vi "AB_Engine_Detect_Additional_Dependencies.vi"(1 "ContextForBuild in":refnum<vi>, 5 "collect dependencies?":bool, 9 "Dependencies in":T1[](array[typedef]), 11 "error in (no error)":errorcluster) -> (10 "Dependencies out":T1[](array[typedef]), 15 "error out":errorcluster)   [LabVIEW 2020]
uses:
  <vilib>/AppBuilder/AB_Dependency.ctl
  <vilib>/Utility/lvfile.llb/LVFileType.ctl
  <vilib>/Utility/lvfile.llb/NI_FileType.lvlib
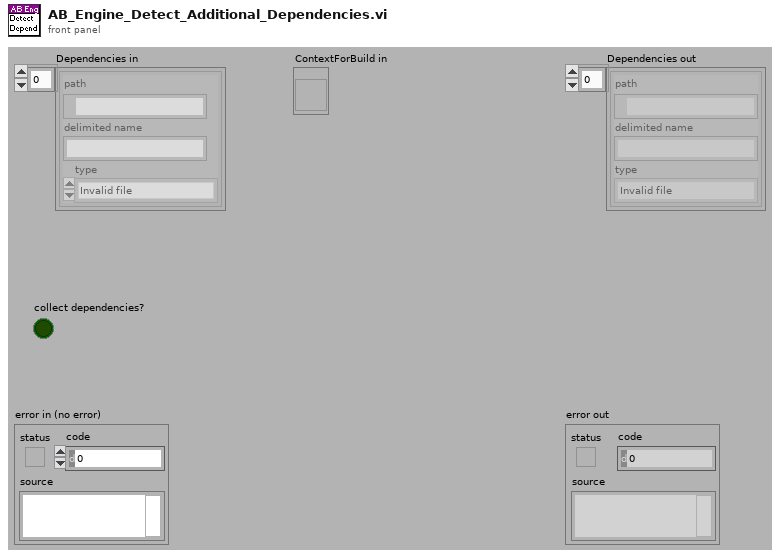
[diagram p1: front panel]
types:
  T1 = typedef "AB_Dependency.ctl" = cluster{"path":path, "delimited name":string, "type":T2}
  T2 = typedef "NI_FileType.lvlib/LVFileType.ctl" = enum32{"Invalid file", "Unknown type", "Instrument", "Control", "Polymorphic VI", "Project", "Library", "LVClass", "XControl", "XNode", "Shared library", ".NET assembly", "ActiveX interface", "CIN", "Run-time menu", "Palette menu", "Help file", "LLB", "XNode Edit Dependency", "Class Private Data Control", "Statechart", "MathScript .m file", "Ladder Diagram", "LVLibp", "XNode Build Dependency"}
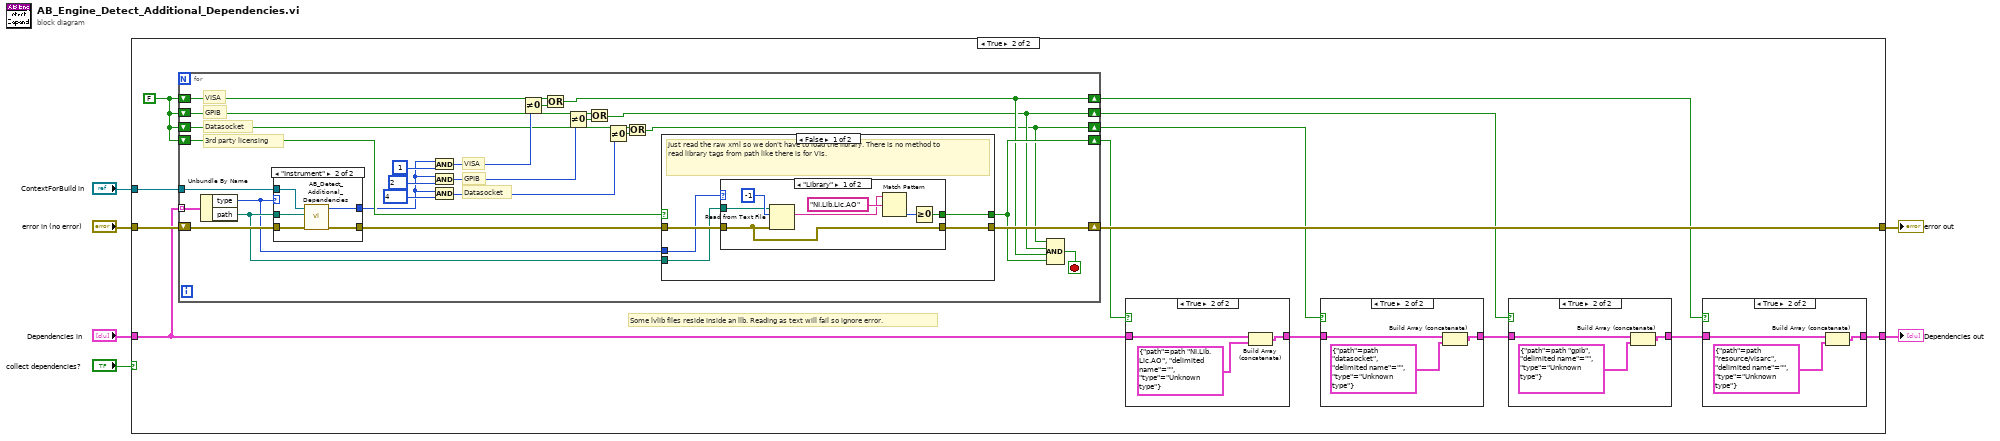
[diagram p0: block diagram]
diagram:
  n1 = case shown="True" "collect dependencies?" {
    tunnel: [w7 w21] -> w5
    tunnel: [w8 w10] -> w4
    tunnel: "error in (no error)" -> [w7 w20]
    tunnel: "Dependencies in" -> [w8 w9]
    tunnel: "ContextForBuild in" -> [_ w17]
    frame False {
    }
    frame True {
      w14 = FALSE ("GPIB detected?")
      # "Some lvlib files reside inside an llb. Reading as text will fail so ignore error."
      n2 = for {
        shift-right: [w63] -> w21
        shift-left: w20 -> [w59]
        shift-right: [w45] -> w18
        shift-left: w14 -> [w46]
        shift-right: [w61] -> w19
        shift-left: w14 -> [w62]
        tunnel: w17 -> [w57]
        shift-right: [w49] -> w15
        shift-left: w14 -> [w52]
        shift-right: [w41] -> w13
        shift-left: w14 -> [w42]
        tunnel: w9 -> [w40] mode=indexing
        stop <- w60 stop-if-true
        # "Datasocket"
        # "GPIB"
        # "VISA"
        # "Datasocket"
        # "VISA"
        # "GPIB"
        # "3rd party licensing"
        n3 = Unbundle By Name(w40) -> ("type"=w38:T2, "path"=w39:path)
        n4 = case shown="\"Instrument\"" w38 {
          tunnel: [_ w69] -> w53
          tunnel: w57 -> [_ w68]
          tunnel: w59 -> [w64 w67]
          tunnel: [w64 w66] -> w58
          tunnel: w39 -> [_ w65]
          frame Default {
          }
          frame "Instrument" {
            n5 = call <vilib>:"AB_Detect_Additional_Dependencies.vi"("error in (no error)"=w67, "source VI path"=w65, "app reference"=w68) -> ("error out"=w66:errorcluster, "Prim Dep Flags"=w69:u32)  [unwired: 7 in]
          }
        }
        n6 = And(x=w53, y=u32 1) -> (x .and. y?=w50:u32)
        n7 = And(x=w53, y=u32 2) -> (x .and. y?=w47:u32)
        n8 = And(x=w53, y=u32 4) -> (x .and. y?=w43:u32)
        n9 = Not Equal To 0?(x=w50) -> (x != 0?=w51:bool)
        n10 = Or(x=w52, y=w51) -> (x .or. y?=w49:bool)
        n11 = Not Equal To 0?(x=w47) -> (x != 0?=w48:bool)
        n12 = Or(x=w46, y=w48) -> (x .or. y?=w45:bool)
        n13 = Not Equal To 0?(x=w43) -> (x != 0?=w44:bool)
        n14 = Or(x=w42, y=w44) -> (x .or. y?=w41:bool)
        n15 = case shown="False" w62 {
          selector: w62 -> [_ w83]
          tunnel: w58 -> [w74 w84]
          tunnel: [w73 w84] -> w63
          tunnel: [w72 w83] -> w61
          tunnel: w39 -> [w71 _]
          tunnel: w38 -> [w70 _]
          frame False {
            # "Just read the raw xml so we don't have to load the library. There is no method to read library tags from path like there is for VIs."
            n16 = case shown="\"Library\"" w70 {
              tunnel: [w80 _] -> w72
              tunnel: w74 -> [w75 w82]
              tunnel: [w75 w82] -> w73
              tunnel: w71 -> [w76 _]
              frame "Library" {
                n17 = Read from Text File(file (use dialog)=w76, count=-1, error in=w75) -> (text=w78:string)  [unwired: 1 in, 3 out]
                n18 = Match Pattern(string=w78, regular expression="NI.Lib.Lic.AO") -> (offset past match=w77:i32)  [unwired: 1 in, 3 out]
                n19 = Greater Or Equal To 0?(x=w77) -> (x >= 0?=w80:bool)
              }
              frame Default {
              }
            }
          }
          frame True {
          }
        }
        n20 = Compound Arithmetic op=AND(w41, w45, w49, w61) -> (w60:bool)
      }
      n21 = case shown="True" w19 {
        tunnel: w9 -> [w34 w37]
        tunnel: [w34 w35] -> w12
        frame False {
        }
        frame True {
          n22 = Build Array (concatenate)(w37, T1 {"path"=path "NI.Lib.Lic.AO", "delimited name"="", "type"=enum."Unknown type"} ("dependency")) -> (w35:T1[])
        }
      }
      n23 = case shown="True" w13 {
        tunnel: w12 -> [w22 w25]
        tunnel: [w22 w24] -> w11
        frame False {
        }
        frame True {
          n24 = Build Array (concatenate)(w25, T1 {"path"=path "datasocket", "delimited name"="", "type"=enum."Unknown type"} ("dependency")) -> (w24:T1[])
        }
      }
      n25 = case shown="True" w18 {
        tunnel: w11 -> [w30 w33]
        tunnel: [w30 w32] -> w16
        frame False {
        }
        frame True {
          n26 = Build Array (concatenate)(w33, T1 {"path"=path "gpib", "delimited name"="", "type"=enum."Unknown type"} ("dependency")) -> (w32:T1[])
        }
      }
      n27 = case shown="True" w15 {
        tunnel: w16 -> [w26 w29]
        tunnel: [w26 w28] -> w10
        frame False {
        }
        frame True {
          n28 = Build Array (concatenate)(w29, T1 {"path"=path "resource/visarc", "delimited name"="", "type"=enum."Unknown type"} ("dependency")) -> (w28:T1[])
        }
      }
    }
  }
  "error out" <- w5
  "Dependencies out" <- w4
